vi "Set Recording Status Attributes.vi"(0 "logging in":T1, 5 "logging duration":dbl, 9 "status info in":variant, 11 "error in (no error)":errorcluster) -> (4 "logging out":T1, 6 "recording complete":bool, 10 "status info out":variant, 15 "error out":errorcluster)   [LabVIEW 2024, in "DSA_CFG_ACQ.lvlib"]
doc: "Continuous data processing is only done when the data exists AND no error. \n\nAll processes/measurements that need continuous data as input are done here. Waveform conditioning (filtering) and software triggering are two such processes. The order in which these are performed matters because both need continuous data as their inputs. Filtering outputs continuous stream of data while triggering outputs discontinuous blocks of data (one new block per detected trigger). Therefore, Filter is applied before Trigger Detection. \n\nAfter filtering and triggering are applied on the acquired data, data is stored into 'Block Data' queue. Note that 'Block Data' queue is a single-element queue. Use lossy enqueue element; the old time domain signal is overwritten by the new time domain signal. enqueue element would block the continuous processing loop until 'Block data' queue was emptied by BLOCK PROCESSING."
uses:
  DSA_CFG_ACQ.lvlib
  controls/SFPLogging Info.ctl
  Dynamic Signal Acquisition (Interactive).lvlib
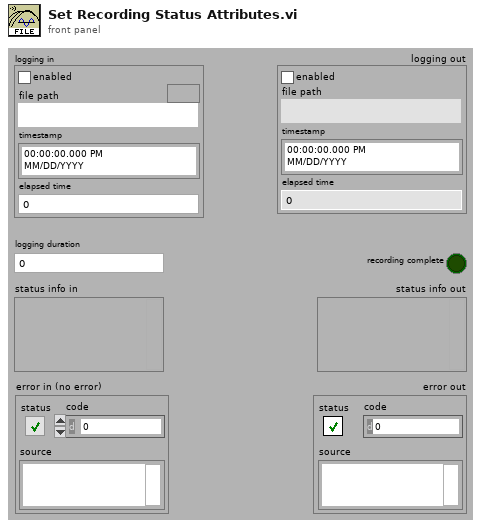
[diagram p1: front panel]
types:
  T1 = typedef "Dynamic Signal Acquisition (Interactive).lvlib/SFPLogging Info.ctl" = cluster{"enabled":bool, "file path":path, "timestamp":timestamp, "elapsed time":dbl}
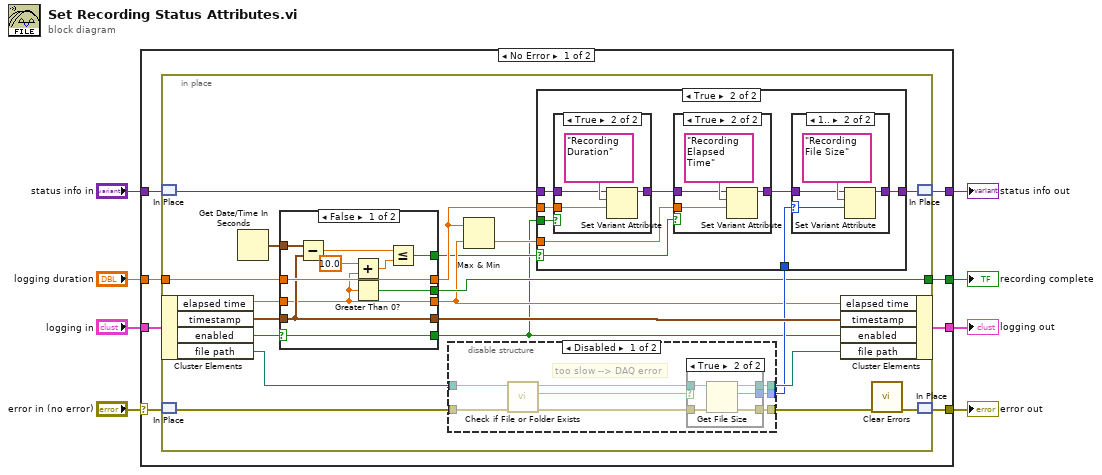
[diagram p0: block diagram]
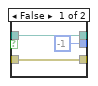
[diagram p2: hidden frame]
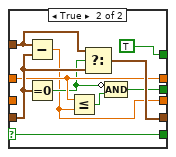
[diagram p8: hidden frame]
diagram:
  n1 = case shown="No Error" "error in (no error)" {
    selector: "error in (no error)" -> [w14 w101]
    tunnel: [w10 w101] -> w8
    tunnel: [w11 w100] -> w6
    tunnel: "status info in" -> [w12 w100]
    tunnel: "logging in" -> [w15 w99]
    tunnel: "logging duration" -> [w16 _]
    tunnel: [w13 w99] -> w2
    tunnel: [w9 _] -> w1
    frame No Error {
      n2 = in-place {
        in-place-border: w16 -> [w29]
        in-place-border: [w30] -> w9
        n3 = in-place-match #1(w12) -> (w33:variant)
        n4 = in-place-cluster #2(w15) -> ("elapsed time"=w24:dbl, "timestamp"=w36:timestamp, "enabled"=w21:bool, "file path"=w18:path)
        n5 = in-place-match #3(w14) -> (w17:errorcluster)
        n6 = Get Date/Time In Seconds() -> (seconds since 1Jan1904=w25:timestamp)
        n7 = case shown="False" w21 {
          selector: w21 -> [w88 w92]
          tunnel: w36 -> [w85 w96]
          tunnel: w29 -> [w87 w95]
          tunnel: [w88 w92] -> w19
          tunnel: [w85 w98] -> w34
          tunnel: [w80 w89] -> w23
          tunnel: [w79 w97] -> w30
          tunnel: [w87 w95] -> w28
          tunnel: w25 -> [w86 w93]
          tunnel: w24 -> [w80 _]
          tunnel: [w84 TRUE] -> w22
          frame False {
            n8 = Subtract(x=w86, y=w85) -> (x-y=w83:dbl)
            n9 = Add(x=10.0, y=w80) -> (x+y=w82:dbl)
            n10 = Greater Than 0?(x=w80) -> (x > 0?=w79:bool)
            n11 = Less Or Equal?(x=w83, y=w82) -> (x <= y?=w84:bool)
          }
          frame True {
            n12 = Subtract(x=w93, y=w96) -> (x-y=w89:dbl)
            n13 = Equal To 0?(x=w96) -> (x = 0?=w91:bool)
            n14 = Less Or Equal?(x=w95, y=w89) -> (x <= y?=w90:bool)
            n15 = Select(t=w93, s=w91, f=w96) -> (s? t:f=w98:timestamp)
            n16 = Compound Arithmetic op=AND(invert w91, w90) -> (w97:bool)
          }
        }
        n17 = disable-structure shown="Disabled" {
          disable-tunnel: w18 -> [w39 w53]
          disable-tunnel: w17 -> [w40 w52]
          disable-tunnel: [w44 w53] -> w35
          disable-tunnel: [w43 _] -> w32
          disable-tunnel: [w42 w52] -> w26
          frame Disabled {
            # "too slow --> DAQ error"
            n18 = call <vilib>:"Check if File or Folder Exists.vi"("error in (no error)"=w40, "path"=w39) -> ("error out"=w37:errorcluster, "file or folder exists?"=w41:bool, "dup path"=w38:path)  [unwired: 7 in]
            n19 = case shown="True" w41 {
              tunnel: w38 -> [w47 w50]
              tunnel: w37 -> [w46 w51]
              tunnel: [w47 w50] -> w44
              tunnel: [w46 w49] -> w42
              tunnel: [i64 -1 ("size (in bytes)") w48] -> w43
              frame False {
              }
              frame True {
                n20 = Get File Size(file=w50, error in=w51) -> (size (in bytes)=w48:i64, 0:w49:errorcluster)  [unwired: 1 out]
              }
            }
          }
          frame Enabled {
          }
        }
        n21 = Max & Min(x=w28, y=w23) -> (min(x,y)=w20:dbl)  [unwired: 1 out]
        n22 = case shown="True" w22 {
          selector: w22 -> [_ w55]
          tunnel: w33 -> [w54 w63]
          tunnel: w19 -> [_ w62]
          tunnel: w32 -> [_ w59]
          tunnel: [w54 w58] -> w31
          tunnel: w20 -> [_ w57]
          tunnel: w28 -> [_ w56]
          frame False {
          }
          frame True {
            n23 = case shown="True" w62 {
              tunnel: w63 -> [w74 w77]
              tunnel: w56 -> [_ w76]
              tunnel: [w74 w75] -> w61
              frame False {
              }
              frame True {
                n24 = Set Variant Attribute(Variant=w77, name="Recording Duration", value=w76) -> (Variant out=w75:variant)  [unwired: 1 in, 2 out]
              }
            }
            n25 = case shown="True" w55 {
              tunnel: w61 -> [w69 w72]
              tunnel: w57 -> [_ w71]
              tunnel: [w69 w70] -> w60
              frame False {
              }
              frame True {
                n26 = Set Variant Attribute(Variant=w72, name="Recording Elapsed Time", value=w71) -> (Variant out=w70:variant)  [unwired: 1 in, 2 out]
              }
            }
            n27 = case shown="1.." w59 {
              selector: w59 -> [_ w65]
              tunnel: w60 -> [w64 w67]
              tunnel: [w64 w66] -> w58
              frame 0, Default {
              }
              frame 1.. {
                n28 = Set Variant Attribute(Variant=w67, name="Recording File Size", value=w65) -> (Variant out=w66:variant)  [unwired: 1 in, 2 out]
              }
            }
          }
        }
        n29 = in-place-cluster #2("elapsed time"=w23, "timestamp"=w34, "enabled"=w19, "file path"=w35) -> (w13:T1)
        n30 = call <vilib>:"Clear Errors.vi"("error in (no error)"=w26) -> ("error out"=w27:errorcluster)  [unwired: 5 in, 1 out]
        n31 = in-place-match #1(w31) -> (w11:variant)
        n32 = in-place-match #3(w27) -> (w10:errorcluster)
      }
    }
    frame Error {
    }
  }
  "error out" <- w8
  "status info out" <- w6
  "logging out" <- w2
  "recording complete" <- w1
